vi "Signal Production.vi"(11 "Polarization":dbl=0.45 min=0.0 max=0.999 step=0.01) -> (3 "output cluster":cluster{dbl[], "result":dbl[]})   [LabVIEW 2019]
panel:
  out "Graph":cluster{dbl[], dbl[]}(graph)
  in  "Squared Lorentzian Width":dbl=0.005 min=0.0 step=0.0001
  in  "eta*cosphi":dbl=-0.0303 step=0.0001
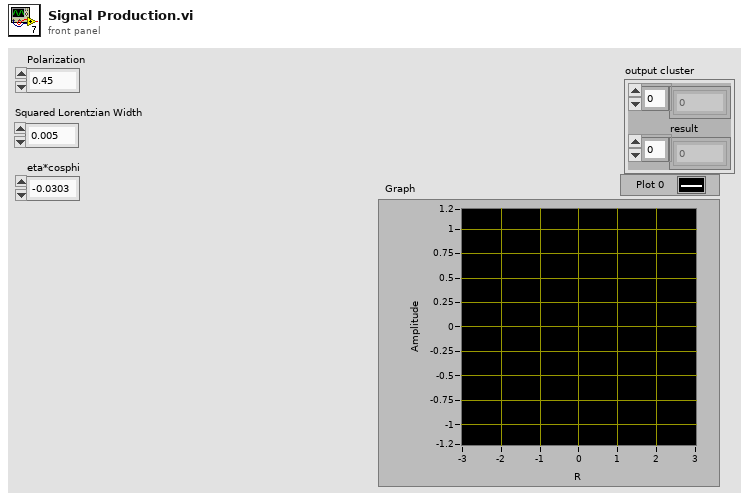
[diagram p1: front panel]
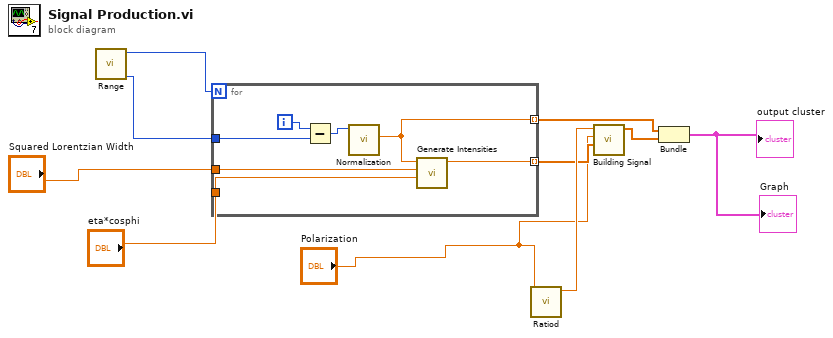
[diagram p0: block diagram]
diagram:
  n1 = call "Range.vi"() -> ("Center"=w3:i32, "NumBins"=w2:i32)  [unwired: 10 in]
  n2 = for {
    N: w2 -> [_]
    tunnel: "Squared Lorentzian Width" -> [w15]
    tunnel: "eta*cosphi" -> [w14]
    tunnel: [w13] -> w9 mode=indexing
    tunnel: [w12] -> w7 mode=indexing
    tunnel: w3 -> [w11]
    i -> [w17]
    n3 = Subtract(x=w17, y=w11) -> (x-y=w16:i32)
    n4 = call "Normalization.vi"("x"=w16) -> ("Normalization"=w12:dbl)  [unwired: 10 in]
    n5 = call "Generate Intensities.vi"("eta*cosalpha"=w14, "Lorentzian Width"=w15, "R"=w12) -> ("Intensity"=w13:dbl)  [unwired: 8 in]
  }
  n6 = call "Ratiod.vi"("P"="Polarization") -> ("r"=w10:dbl)  [unwired: 10 in]
  n7 = call "Building Signal.vi"("I array in"=w9, "Polarization"="Polarization", "Ratio"=w10) -> ("result"=w8:dbl[])  [unwired: 8 in]
  n8 = Bundle(w7, "result"=w8) -> (→"output cluster" →"Graph":cluster{dbl[], "result":dbl[]})  [unwired: 1 in]
